vi "Write Row.vi"(8 "error in (no error)":errorcluster, 10 "Row":refnum<k24>, 11 "UserAddedRow in":refnum<class "UserDeletedRow.lvclass">) -> (0 "error out":errorcluster, 3 "UserAddedRow out":refnum<class "UserDeletedRow.lvclass">)   [LabVIEW 2016, in "DataGrid.lvlib" / "UserDeletedRow.lvclass"]
uses:
  <userlib>/LabVIEWdotNetDataGrid/source/Events/UserDeletedRow/UserDeletedRow.lvclass
  System.Windows.Forms
  <userlib>/LabVIEWdotNetDataGrid/source/Events/UserDeletedRow/UserDeletedRow.lvclass/UserDeletedRow.ctl
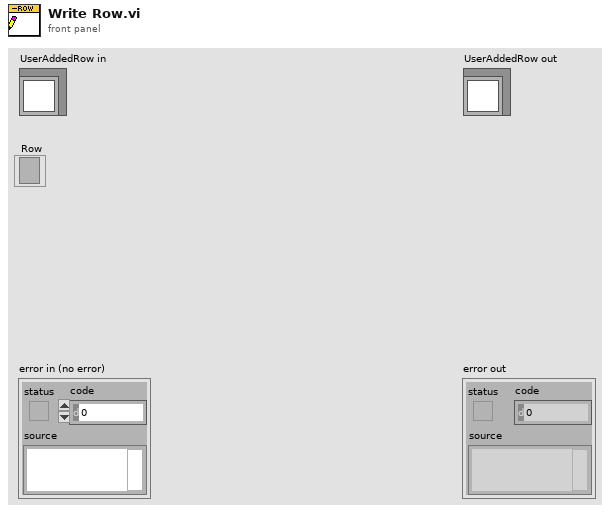
[diagram p1: front panel]
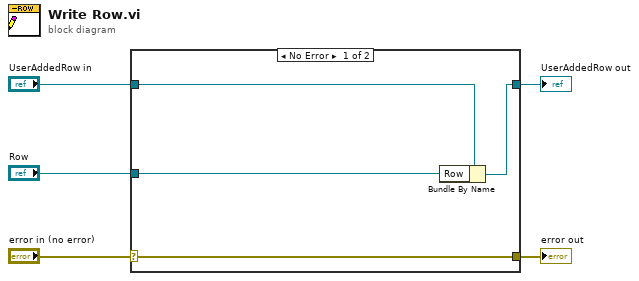
[diagram p0: block diagram]
diagram:
  n1 = case shown="No Error" "error in (no error)" {
    selector: "error in (no error)" -> [w9 w10]
    tunnel: [w9 w10] -> w4
    tunnel: [w7 w11] -> w2
    tunnel: "UserAddedRow in" -> [w8 w11]
    tunnel: "Row" -> [w6 _]
    frame No Error {
      n2 = Bundle By Name(cluster=w8, "Row"=w6) -> (w7:refnum<class "UserDeletedRow.lvclass">)
    }
    frame Error {
    }
  }
  "error out" <- w4
  "UserAddedRow out" <- w2
